vi "dashboard.vi"() -> ()   [LabVIEW 2025]
panel:
  out "Waveform Chart":cluster{dbl, dbl}(graph)
  out "measured_angle":dbl
  in  "kd":string
  in  "ki":string
  in  "kp":string
  in  "target_angle":string
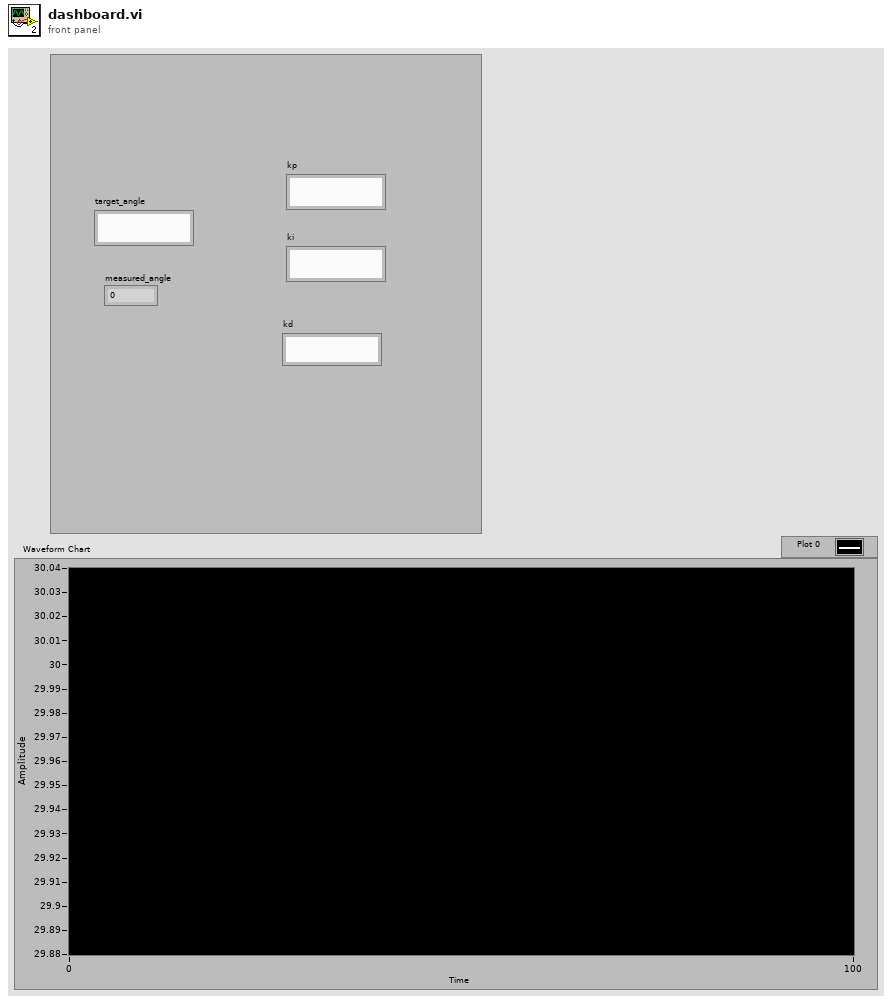
[diagram p1: front panel]
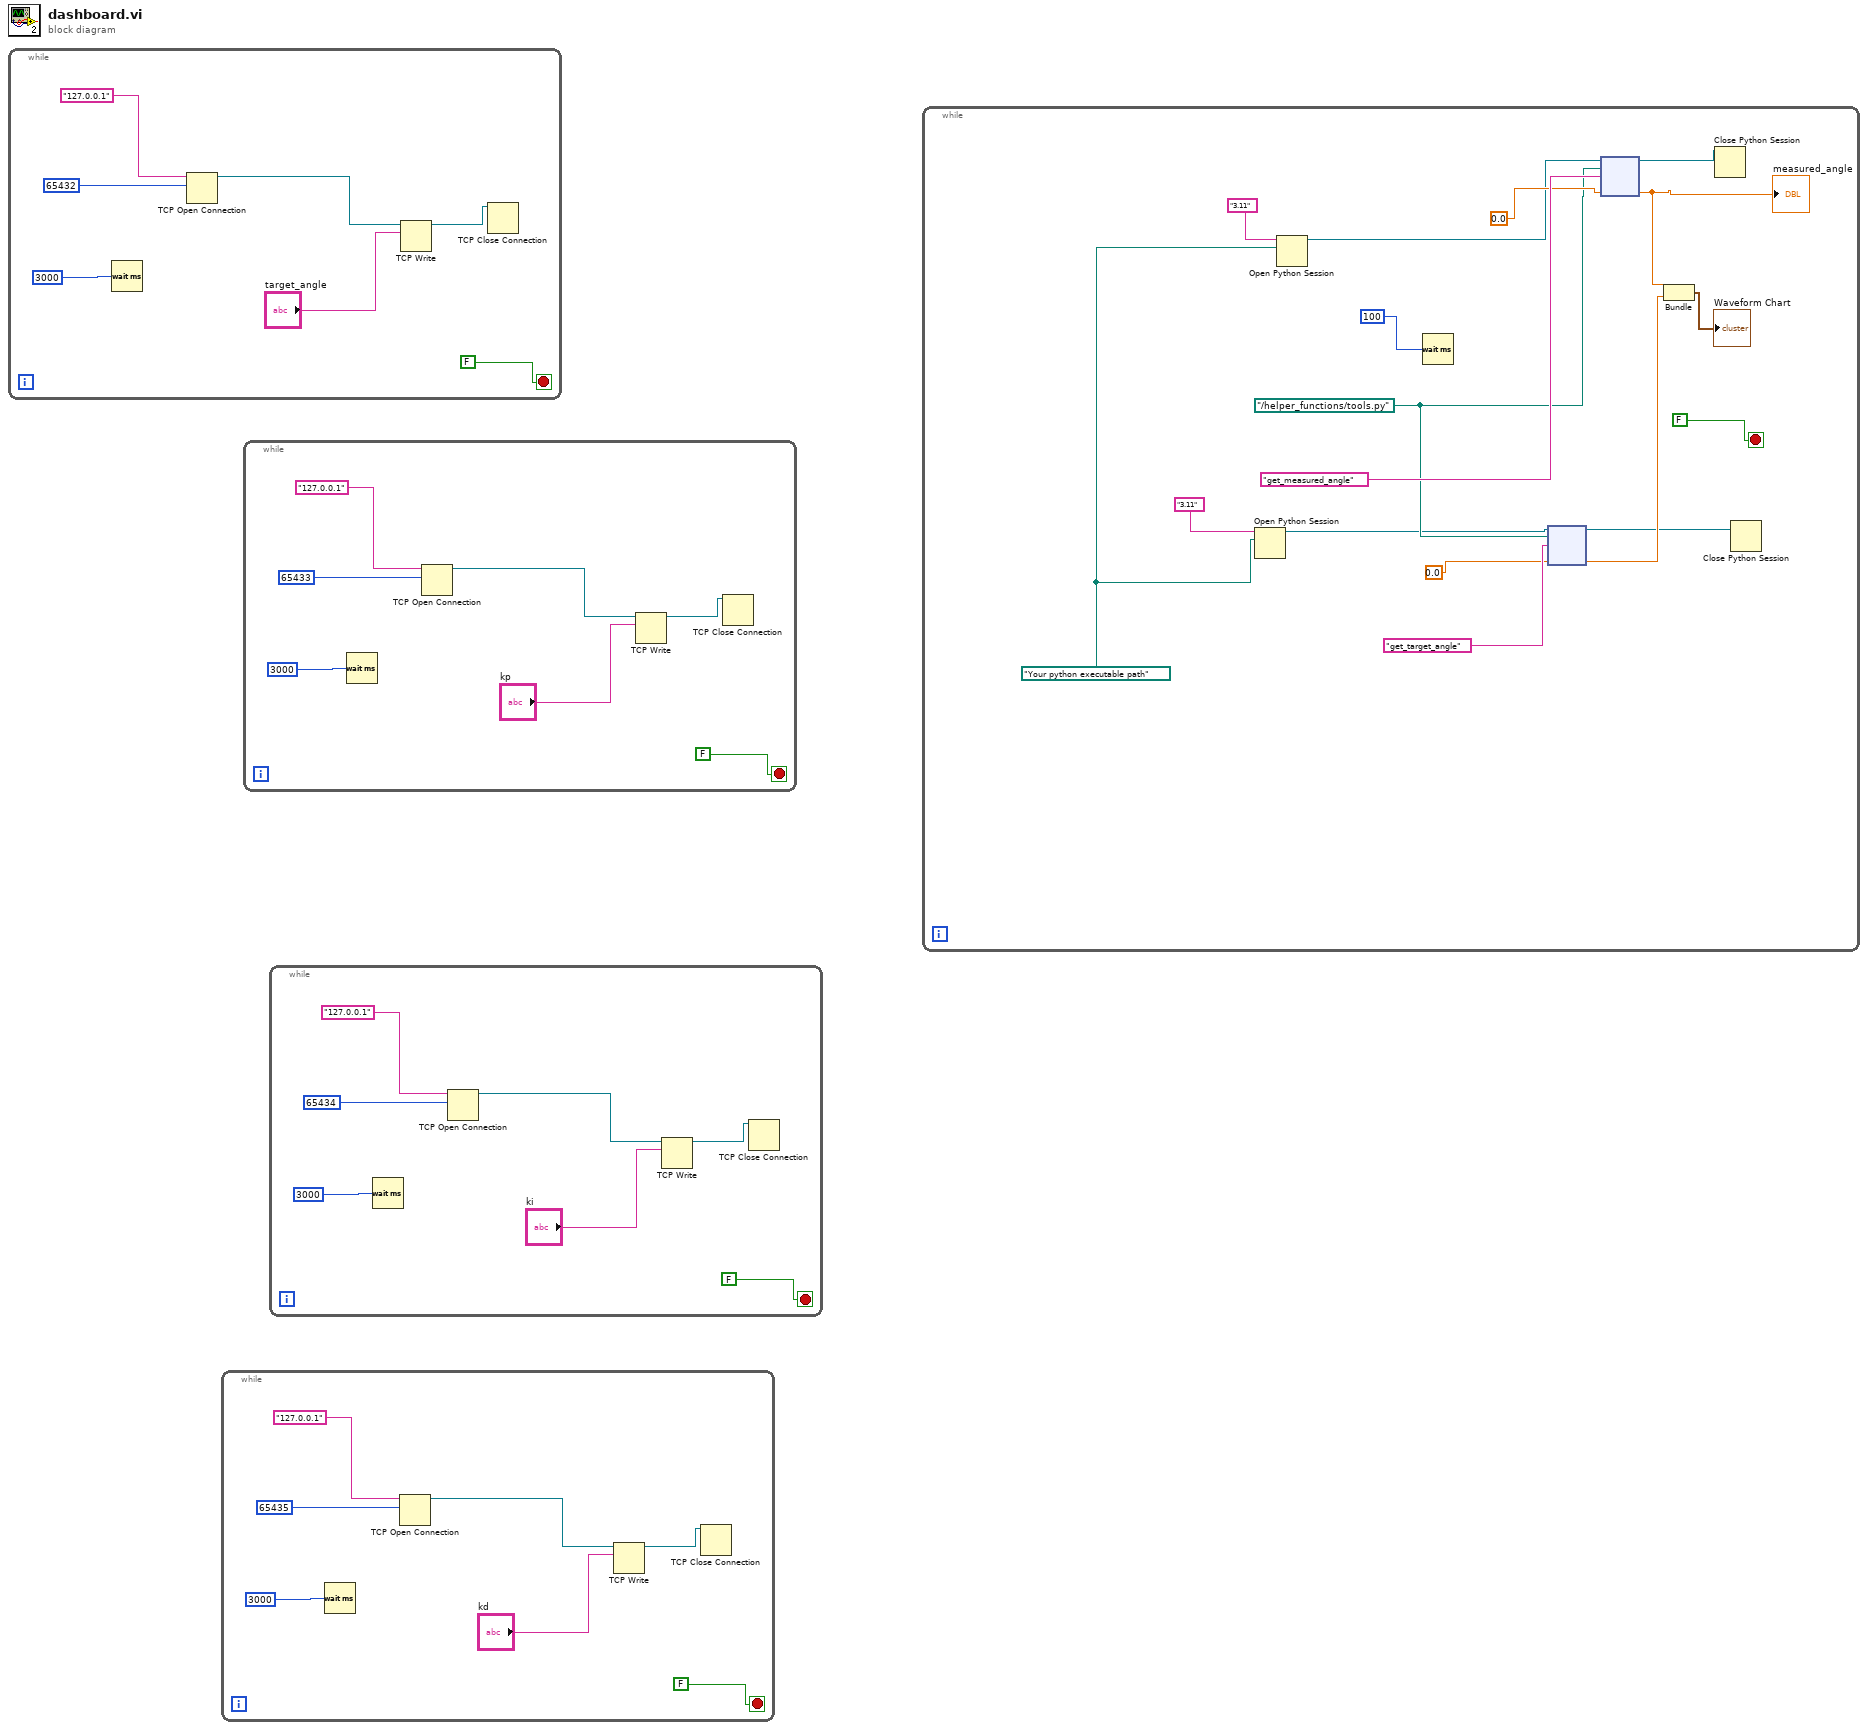
[diagram p0: block diagram]
diagram:
  n1 = while {
    stop <- FALSE stop-if-true
    n2 = Wait (ms)(milliseconds to wait=3000) -> ()  [unwired: 1 out]
    n3 = TCP Open Connection(address="127.0.0.1", remote port or service name=u16 65432) -> (connection ID=w5:refnum<k5>)  [unwired: 3 in, 1 out]
    n4 = TCP Write(connection ID=w5, data in="target_angle") -> (connection ID out=w3:refnum<k5>)  [unwired: 2 in, 2 out]
    n5 = TCP Close Connection(connection ID=w3) -> ()  [unwired: 2 in, 2 out]
  }
  n6 = while {
    stop <- FALSE stop-if-true
    n7 = Wait (ms)(milliseconds to wait=3000) -> ()  [unwired: 1 out]
    n8 = TCP Open Connection(address="127.0.0.1", remote port or service name=u16 65435) -> (connection ID=w12:refnum<k5>)  [unwired: 3 in, 1 out]
    n9 = TCP Write(connection ID=w12, data in="kd") -> (connection ID out=w10:refnum<k5>)  [unwired: 2 in, 2 out]
    n10 = TCP Close Connection(connection ID=w10) -> ()  [unwired: 2 in, 2 out]
  }
  n11 = while {
    stop <- FALSE stop-if-true
    n12 = Wait (ms)(milliseconds to wait=3000) -> ()  [unwired: 1 out]
    n13 = TCP Open Connection(address="127.0.0.1", remote port or service name=u16 65433) -> (connection ID=w19:refnum<k5>)  [unwired: 3 in, 1 out]
    n14 = TCP Write(connection ID=w19, data in="kp") -> (connection ID out=w17:refnum<k5>)  [unwired: 2 in, 2 out]
    n15 = TCP Close Connection(connection ID=w17) -> ()  [unwired: 2 in, 2 out]
  }
  n16 = while {
    stop <- FALSE stop-if-true
    n17 = Wait (ms)(milliseconds to wait=3000) -> ()  [unwired: 1 out]
    n18 = TCP Open Connection(address="127.0.0.1", remote port or service name=u16 65434) -> (connection ID=w26:refnum<k5>)  [unwired: 3 in, 1 out]
    n19 = TCP Write(connection ID=w26, data in="ki") -> (connection ID out=w24:refnum<k5>)  [unwired: 2 in, 2 out]
    n20 = TCP Close Connection(connection ID=w24) -> ()  [unwired: 2 in, 2 out]
  }
  n21 = while {
    stop <- FALSE stop-if-true
    w29 = path "Your python executable path" ("Python path")
    w35 = path "../helper_functions/tools.py" ("module path")
    n22 = Open Python Session(python version="3.11" ("Python version"), python path=w29) -> (session out=w32:refnum<k35>)  [unwired: 1 in, 1 out]
    n23 = Open Python Session(python version="3.11" ("Python version"), python path=w29) -> (session out=w37:refnum<k35>)  [unwired: 1 in, 1 out]
    n24 = Wait (ms)(milliseconds to wait=100) -> ()  [unwired: 1 out]
    n25 = node(w32, w35, "get_target_angle" ("function name"), 0.0) -> (w30:refnum<k35>, w34:dbl)  [unwired: 1 in, 3 out]
    n26 = node(w37, w35, "get_measured_angle" ("function name"), 0.0) -> (w31:refnum<k35>, w40:dbl)  [unwired: 1 in, 3 out]
    "measured_angle" <- w40
    n27 = Bundle(w40, w34) -> (→"Waveform Chart":cluster{dbl, dbl})  [unwired: 1 in]
    n28 = Close Python Session(session in=w31) -> ()  [unwired: 1 in, 1 out]
    n29 = Close Python Session(session in=w30) -> ()  [unwired: 1 in, 1 out]
  }
